vi "sub_Build_Packet.vi"(7 "Sync Sequence Bitstream":i8[](array[numeric]), 8 "Cyclic Padding Bits":i32, 9 "Packet number":i16, 10 "Packet Parameters in":T1={"Length of sync sequence (50)"=50, "Number of message bits"=128, "Number of guardbits"=40, "Sync PN sequence order (31)"=31, "Number of header bits"=16, "Packet Pad [samples]"=0}, 11 "Input Message":i8[](array[numeric])) -> (3 "Packet out":i8[](array[numeric]))   [LabVIEW 2014]
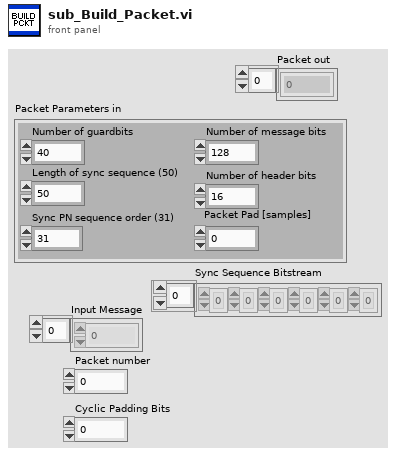
[diagram p1: front panel]
types:
  T1 = cluster{"Length of sync sequence (50)":i32, "Number of message bits":i32, "Number of guardbits":i32, "Sync PN sequence order (31)":i32, "Number of header bits":i32, "Packet Pad [samples]":i32}
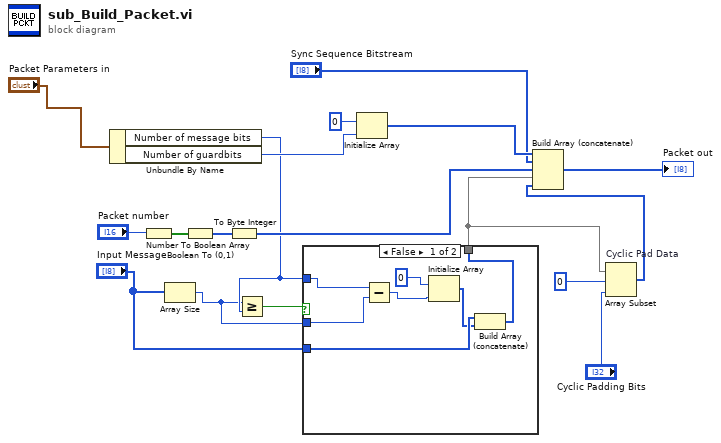
[diagram p0: block diagram]
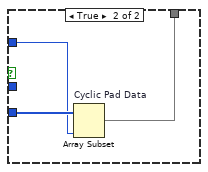
[diagram p2: hidden frame]
diagram:
  n1 = Unbundle By Name("Packet Parameters in") -> ("Number of message bits"=w6:i32, "Number of guardbits"=w17:i32)
  n2 = Number To Boolean Array(number="Packet number") -> (Boolean array=w13:bool[])
  n3 = Array Size(array="Input Message") -> (size(s)=w5:i32)
  n4 = Boolean To (0,1)(Boolean=w13) -> (0, 1=w14:i16[])
  n5 = To Byte Integer(number=w14) -> (8bit integer=w11:i8[])
  n6 = Greater Or Equal?(x=w5, y=w6) -> (x >= y?=w8:bool)
  n7 = case shown="False" w8 {
    tunnel: "Input Message" -> [w21 w28]
    tunnel: w6 -> [w24 w27]
    tunnel: [w19 w26] -> w4
    tunnel: w5 -> [w23 _]
    frame False {
      n8 = Subtract(x=w24, y=w23) -> (x-y=w22:i32)
      n9 = Initialize Array(i8 0, w22) -> (w20:i8[])
      n10 = Build Array (concatenate)(w21, w20) -> (w19:i8[])
    }
    frame True {
      n11 = Array Subset "Cyclic Pad Data"(array=w28, length=w27) -> (w26:i8[])  [unwired: 1 in]
    }
  }
  n12 = Initialize Array(i8 0, w17) -> (w16:i8[])
  n13 = Array Subset "Cyclic Pad Data"(array=w4, index=0, length="Cyclic Padding Bits") -> (w3:i8[])
  n14 = Build Array (concatenate)(w16, "Sync Sequence Bitstream", w11, w4, w3) -> (→"Packet out":i8[])
